vi "FlatToRichnixnet_grpc_DbGetDatabaseListResponse.vi"(5 "OutputClusterType":T1, 11 "InputCluster":T2) -> (3 "OutputCluster":T1)   [LabVIEW 2025, in "grpc-xnet_client.lvlib"]
uses:
  grpc-xnet_client.lvlib
  nixnet_grpc_DbGetDatabaseListResponse_Flat.ctl
  nixnet_grpc_DbGetDatabaseListResponse.ctl
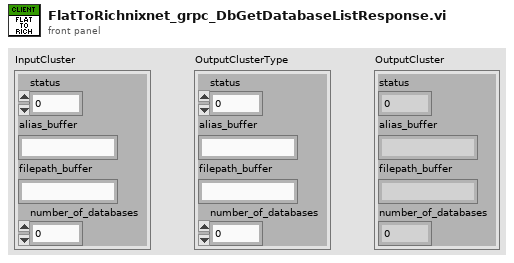
[diagram p1: front panel]
types:
  T1 = typedef "grpc-xnet_client.lvlib/nixnet_grpc_DbGetDatabaseListResponse.ctl" = cluster{"status":i32, "alias_buffer":string, "filepath_buffer":string, "number_of_databases":u32}
  T2 = typedef "grpc-xnet_client.lvlib/nixnet_grpc_DbGetDatabaseListResponse_Flat.ctl" = cluster{"status":i32, "alias_buffer":string, "filepath_buffer":string, "number_of_databases":u32}
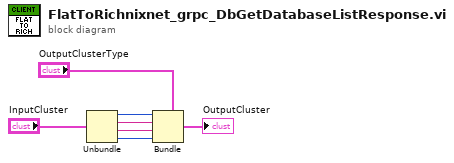
[diagram p0: block diagram]
diagram:
  n1 = Unbundle "Unbundle"("InputCluster") -> ("status"=w4:i32, "alias_buffer"=w3:string, "filepath_buffer"=w2:string, "number_of_databases"=w1:u32)
  n2 = Bundle "Bundle"(cluster="OutputClusterType", "status"=w4, "alias_buffer"=w3, "filepath_buffer"=w2, "number_of_databases"=w1) -> (→"OutputCluster":T1)
